vi "Configure Output.vi"(7 "Enable Output (T: Enable)":bool, 8 "error in (no error)":errorcluster, 10 "Ch Selector":T1, 11 "VISA resource name":refnum<visa-resource-name>) -> (0 "error out":errorcluster, 3 "VISA resource name out":refnum<visa-resource-name>)   [LabVIEW 2020, in "ScientiFic DC Power Supply.lvlib"]
doc: "Configures output voltage level, channel, and enables or disables the output of the power supply."
uses:
  <instrlib>/ScientiFic DC Power Supply/ScientiFic DC Power Supply.lvlib
  <instrlib>/ScientiFic DC Power Supply/Public/Ch Selector.ctl
panel:
  out "concatenated string":string
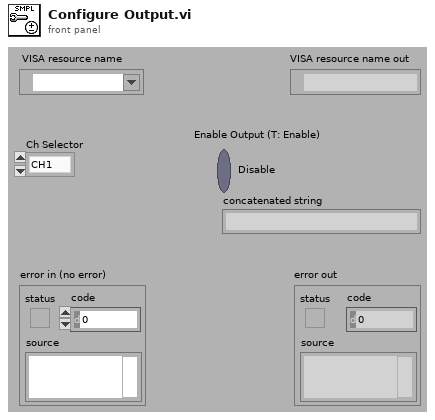
[diagram p1: front panel]
types:
  T1 = typedef "ScientiFic DC Power Supply.lvlib/Ch Selector.ctl" = enum16{"CH1", "CH2", "CH3", "CH4"}
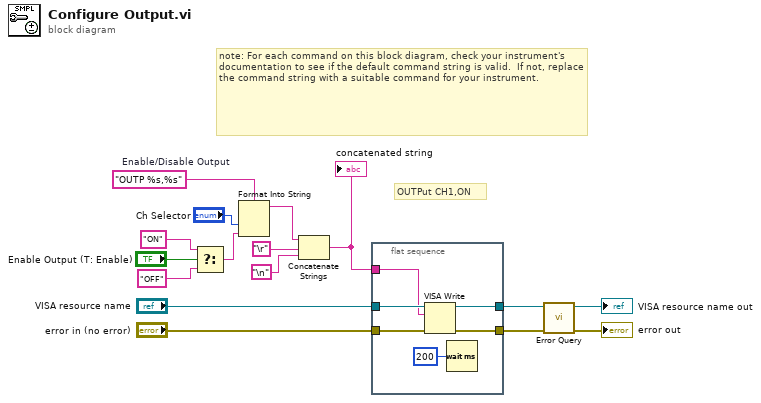
[diagram p0: block diagram]
diagram:
  w14 = "OUTP %s,%s"  # Enable/Disable Output
  # "OUTPut CH1,ON"
  # "note: For each command on this block diagram, check your instrument's documentation to see if the default command string is valid.  If not, replace the command string with a suitable command for your instrument."
  n1 = Select(t="ON", s="Enable Output (T: Enable)", f="OFF") -> (s? t:f=w4:string)
  n2 = Format Into String(format string=w14, "Ch Selector", w4) -> (resulting string=w7:string)  [unwired: 2 in, 1 out]
  n3 = Concatenate Strings(w7, "\r", "\n") -> (w6:string)
  "concatenated string" <- w6
  n4 = flat-sequence {
    tunnel: [w22] -> w13
    tunnel: [w21] -> w12
    tunnel: "VISA resource name" -> [w20]
    tunnel: "error in (no error)" -> [w19]
    tunnel: w6 -> [w18]
    frame #0 {
      n5 = VISA Write(VISA resource name=w20, write buffer=w18, error in (no error)=w19) -> (VISA resource name out=w22:refnum<visa-resource-name>, error out=w21:errorcluster)  [unwired: 1 out]
      n6 = Wait (ms)(milliseconds to wait=u32 200) -> ()  [unwired: 1 out]
    }
  }
  n7 = call <instrlib>:"Error Query.vi"("error in (no error)"=w12, "VISA resource name"=w13) -> ("error out"=→"error out":errorcluster, "VISA resource name out"=→"VISA resource name out":refnum<visa-resource-name>)  [unwired: 8 in]
